vi "Prompt Flatten Test Parameters.vi"(7 "Test Configuration (\"\")":string, 9 "error in (no error)":errorcluster, 10 "Parameter Variant":variant) -> (1 "error out":errorcluster, 2 "Parameter String":string)   [LabVIEW 2011]
uses:
  TypeDefs/Prompt Test Parameters.ctl
  Prompt Version.vi
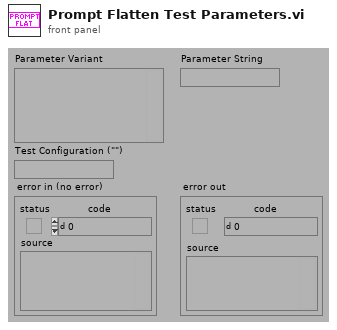
[diagram p1: front panel]
types:
  T1 = typedef "Prompt Test Parameters.ctl" = cluster{"Prompt":string}
  T2 = typedef "OGAB Version.ctl" = cluster{"Version":string, "Build Number":u32, "Build Date/Time":dbl}
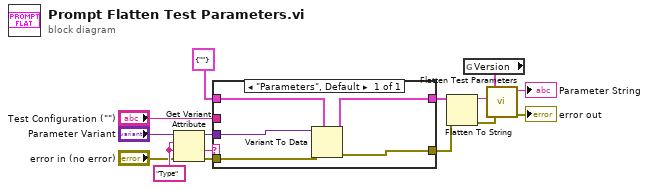
[diagram p0: block diagram]
diagram:
  w14 = "Type" ("name")
  n1 = Get Variant Attribute(Variant="Parameter Variant", name=w14, default value (empty Variant)=w14, error in="error in (no error)") -> (duplicate Variant=w5:variant, value=w1:string, error out=w7:errorcluster)  [unwired: 1 out]
  n2 = case shown="\"Parameters\", Default" w1 {
    tunnel: w5 -> [w20]
    tunnel: T1 {"Prompt"=""} ("Prompt Test Parameters") -> [w16]
    tunnel: [w17] -> w3
    tunnel: [w19] -> w2
    tunnel: w7 -> [w18]
    tunnel: "Test Configuration (\"\")" -> [_]
    frame "Parameters", Default {
      n3 = Variant To Data(error in=w18, type=w16, Variant=w20) -> (data=w17:T1, error out=w19:errorcluster)
    }
  }
  n4 = Flatten To String(anything=w3, error in (no error)=w2) -> (data string=w13:string, error out=w11:errorcluster)  [unwired: 3 out]
  n5 = global read "Prompt Version.vi" "Version"() -> (w12:T2)
  n6 = call "Flatten Test Parameters.vi"("error in (no error)"=w11, "Flattened Test Parameters (\"\")"=w13, "Test Version"=w12) -> ("error out"=→"error out":errorcluster, "Flattened Test Parameters with Version"=→"Parameter String":string)  [unwired: 3 out]
